vi "Wake Up.vi"(8 "error in (no error)":errorcluster, 11 "Baby in":refnum<class "Baby.lvclass">) -> (0 "error out":errorcluster, 3 "Baby out":refnum<class "Baby.lvclass">)   [LabVIEW 2009, in "Baby.lvclass"]
doc: "Provides a method for the ISleepable Interface to wake up the baby without pinching her."
uses:
  Baby.lvclass
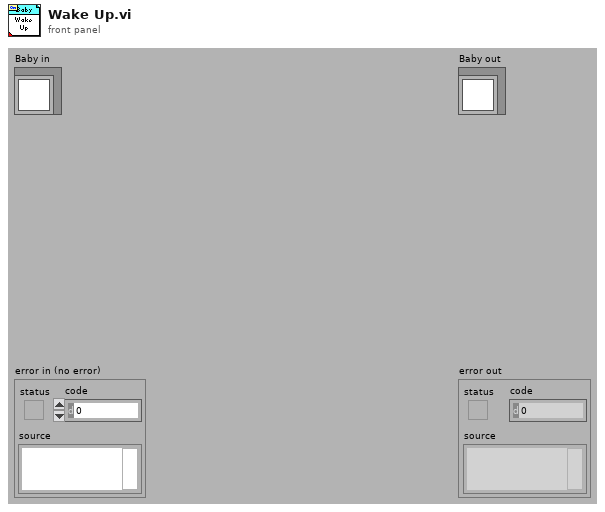
[diagram p1: front panel]
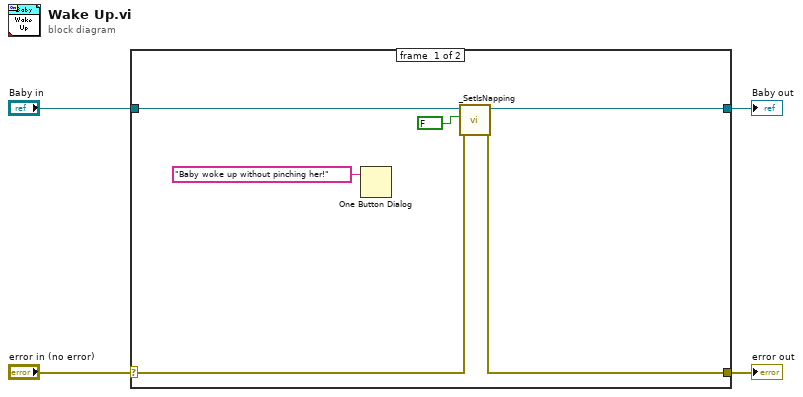
[diagram p0: block diagram]
diagram:
  n1 = case shown="No Error" "error in (no error)" {
    selector: "error in (no error)" -> [w6 w12]
    tunnel: [w5 w12] -> w3
    tunnel: [w9 w11] -> w1
    tunnel: "Baby in" -> [w8 w11]
    frame #0 {
      n2 = One Button Dialog(message="Baby woke up without pinching her!") -> ()  [unwired: 1 in, 1 out]
      n3 = call "_SetIsNapping.vi"("error in (no error)"=w6, "IsNapping (F)"=FALSE ("IsAsleep"), "Baby in"=w8) -> ("error out"=w5:errorcluster, "Baby out"=w9:refnum<class "Baby.lvclass">)  [unwired: 7 in]
    }
    frame #1 {
    }
  }
  "error out" <- w3
  "Baby out" <- w1
